vi "controlLaw_Integral_trackTraj.vi"(7 "ControlParams":T1={"umax"=3.0, "y_ref(k)"=0.0, "Ki"=0.0, "y(k) (from plant)"=0.0, "ND"=0, "NS"=0, "u_Kx_ref(k)"=0.0, "du_max"=3.0, "NS_obs"=0, "NS_control"=0} {"du_max" format="%#_13g"; "u_Kx_ref(k)" format="%#_13g"; "Ki" format="%#_13g"; "y_ref(k)" format="%#_13g"; "umax" format="%#_13g"}, 8 "x^(k)":sgl[](array[numeric])=[0.0, 0.0, 0.0, 0.0, 0.0, 0.0, 0.0, 0.0, 0.0, 0.0, 0.0, 0.0, 0.0, 0.0, 0.0, 0.0, 0.0, 0.0, 0.0, 0.0, 0.0, 0.0, 0.0, 0.0, 0.0]) -> (0 "x^(k+1) = Ax + Bu + Lye":sgl[](array[numeric]), 3 "u(k) (saturated)":sgl)   [LabVIEW 2017]
uses:
  controls/controlParams_tracktraj.ctl
  <vilib>/Platform/TimedLoop/XDataNode/timing_clust.ctl
  <vilib>/Platform/TimedLoop/XDataNode/nitl_modes.ctl
  <vilib>/Platform/TimedLoop/XDataNode/wakeup.ctl
  <vilib>/rvi/DataTransferAndStorage/Container/Common/niFpgaContainerExecOnDevCompGetState.vi
  <vilib>/rvi/Emulation/niFpgaEmulationIsFPGAContextNoSignature.vi
  <vilib>/rvi/DataTransferAndStorage/Container/Common/niFpgaContainerGetUniqueNameForEmu.vi
  <vilib>/rvi/Memory/Memory_Emulation/niFpgaMemoryEmulationCacheClearOnFirstRun.vi
  <vilib>/rvi/Memory/Memory_Emulation/nirvimemoryEmulationManagerCache_MakeExclusive.vi
  <vilib>/rvi/Memory/Memory_Emulation/niFpgaMemoryEmulationValidateCache.vi
  <vilib>/rvi/Memory/Memory_Emulation/nirvimemoryEmulationManagerCache_InsertValue.vi
  <vilib>/Utility/error.llb/Clear Errors.vi
  <vilib>/rvi/Memory/Memory_Emulation/nirvimemoryEmulationManagerCache_ReleaseExclusive.vi
  <vilib>/rvi/Memory/Memory_Emulation/nirvimemoryEmulationManagerCache_GetValue.vi
  <vilib>/rvi/Memory/Memory_Emulation/nirvimemoryEmulationManagerCache_SetValue.vi
  <vilib>/rvi/Emulation/niFpgaProcessEmulError.vi
  <vilib>/rvi/Emulation/niFpgaSctlEmulationGetInTimedLoop.vi
  <vilib>/rvi/Emulation/niFpgaEmulationReportErrorSimple.vi
  <vilib>/rvi/Emulation/niFpgaGetClockAttributes.vi
  <vilib>/rvi/Emulation/niFpgaCriticalErrorInLSC.vi
  <vilib>/Platform/TimedLoop/XDataNode/XDataNode.xnode
  <vilib>/rvi/DataTransferAndStorage/Container/XNode/niFpgaContainer.xnode
  <vilib>/rvi/DataTransferAndStorage/Register/Emulation/niFpgaRegisterEmulationRefIn.vi
  <vilib>/Platform/TimedLoop/XDataNode/XDNodeRunTimeDep.lvlib
panel:
  out "u = -Kx + Nbar*r":sgl format="%#_13g"
  out "-K*x(k)":sgl format="%#_13g"
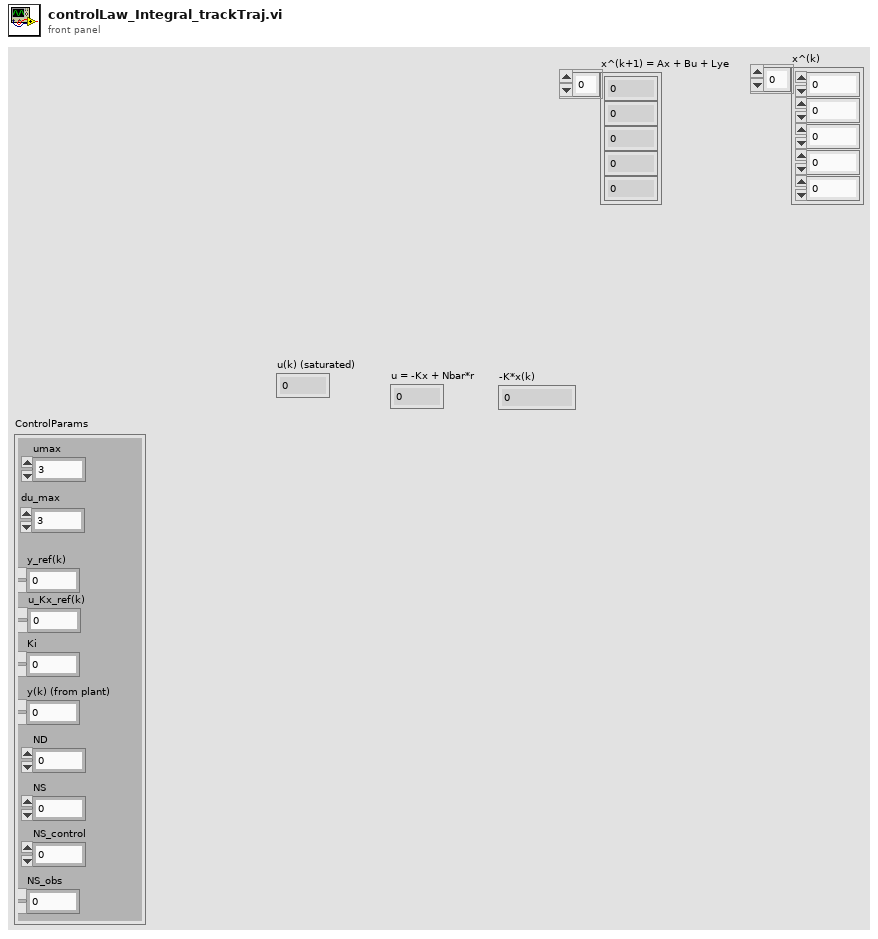
[diagram p1: front panel]
types:
  T1 = typedef "controlParams_tracktraj.ctl" = cluster{"umax":sgl, "y_ref(k)":sgl, "Ki":sgl, "y(k) (from plant)":sgl, "ND":i16, "NS":i16, "u_Kx_ref(k)":sgl, "du_max":sgl, "NS_obs":i16, "NS_control":i16}
  T2 = typedef "XDNodeRunTimeDep.lvlib/timing_clust.ctl" = cluster{"Expected End [f-1]":u64, "Actual End [f-1]":u64, "Finished Late? [f-1]":bool, "Expected End [i-1]":u64, "Actual End [i-1]":u64, "Finished Late? [i-1]":bool, "Expected Start [i]":u64, "Actual Start [i]":u64, "Expected Start [f]":u64, "Actual Start [f]":u64, "Source Name":string, "Structure Name":string, "Period":i64, "Deadline":i64, "Offset":i64, "Start":i64, "Priority":i32, "Timeout":i32, "Mode":T3, "Wakeup Reason":T4, "Error":errorcluster, "Source Type":string, "Secondary Source Type":string, "Global End Time":u64, "Global Start Time":u64, "Frame Duration":u64, "Iteration Duration":u64, "Assigned CPU":i32, "I/O Scan Engine Mode":u32}
  T3 = typedef "XDNodeRunTimeDep.lvlib/nitl_modes.ctl" = enum32{"No Change", "Process missed periods, maintain original phase", "Discard missed periods, maintain original phase", "Process missed periods, ignore original phase", "Discard missed periods, ignore original phase"}
  T4 = typedef "XDNodeRunTimeDep.lvlib/wakeup.ctl" = enum32{"Normal", "Aborted", "Asynchronous wakeup", "Timing source error", "Timed loop error", "Timeout"}
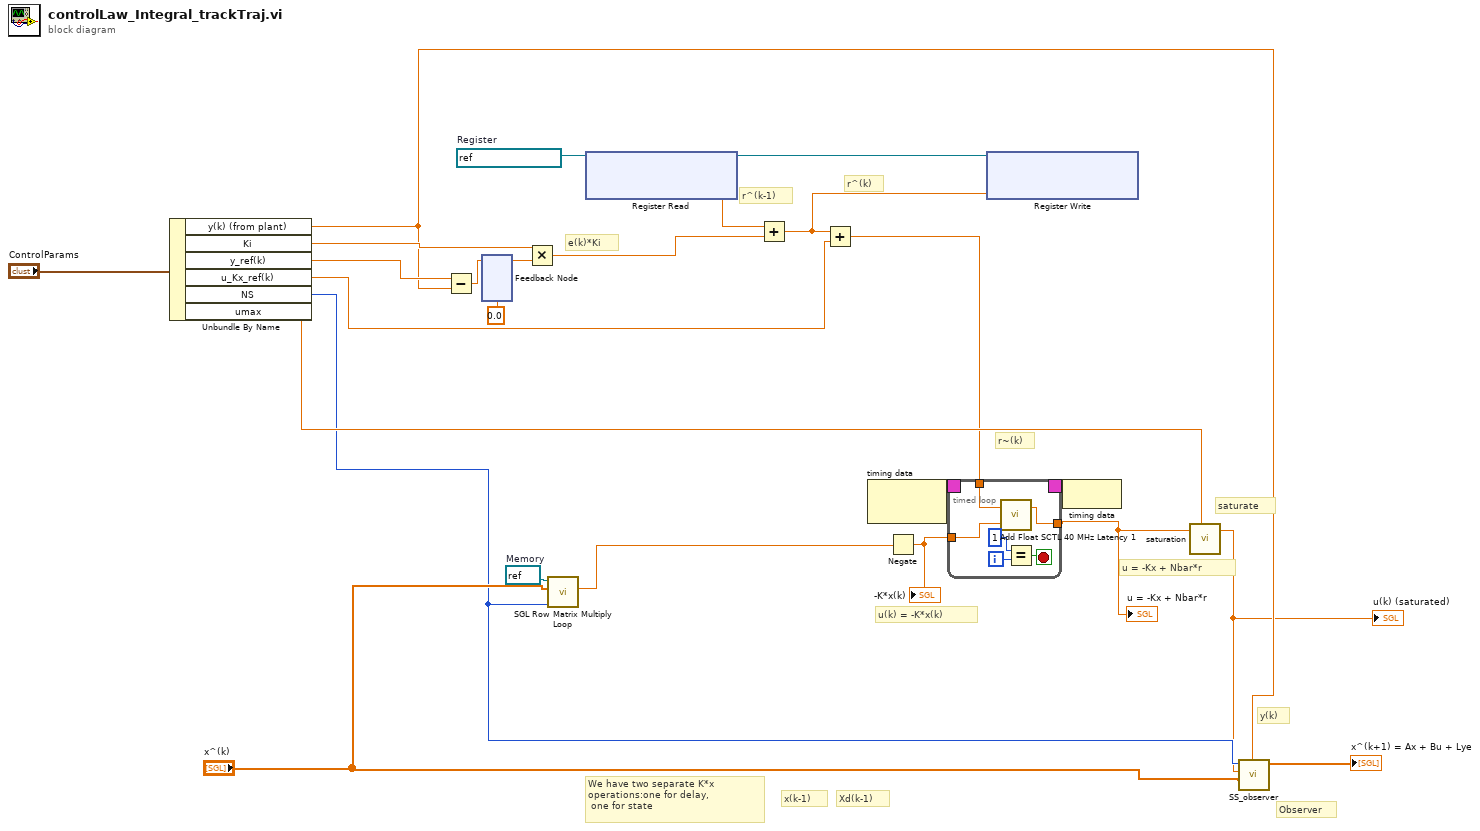
[diagram p0: block diagram]
diagram:
  w16 = refnum<k21> "accumulator"  # Register
  w21 = refnum<k21> "K"  # Memory
  # "y(k)"
  # "Xd(k-1)"
  # "x(k-1)"
  # "r^(k)"
  # "r^(k-1)"
  # "e(k)*Ki"
  # "r~(k)"
  # "We have two separate K*x\noperations:one for delay,\n one for state"
  # "saturate"
  # "u = -Kx + Nbar*r"
  # "u(k) = -K*x(k)"
  # "Observer"
  n1 = Unbundle By Name("ControlParams") -> ("y(k) (from plant)"=w7:sgl, "Ki"=w15:sgl, "y_ref(k)"=w14:sgl, "u_Kx_ref(k)"=w9:sgl, "NS"=w4:i16, "umax"=w13:sgl)
  n2 = Subtract(x=w14, y=w7) -> (x-y=w11:sgl)
  n3 = feedback #1(sgl 0.0) -> (w12:sgl)
  n4 = feedback-in #1(w11) -> ()
  n5 = Multiply(x=w15, y=w12) -> (x*y=w18:sgl)
  n6 = call "SGL Row Matrix Multiply Loop.vi"("NS"=w4, "X"="x^(k)", "Refnum in"=w21) -> ("Numeric"=w2:sgl)  [unwired: 8 in]
  n7 = xnode ("Register Read")("Register In"=w16) -> ("Data"=w19:sgl, "Register Out"=w20:refnum<k21>)
  n8 = Add(x=w19, y=w18) -> (x+y=w17:sgl)
  n9 = Add(x=w17, y=w9) -> (x+y=w8:sgl)
  n10 = node-c288() -> (w25:T2)  [unwired: 1 in]
  n11 = Negate(x=w2) -> (-x=w22:sgl)
  "-K*x(k)" <- w22
  n12 = timed-loop {
    timing: w25 -> [_]
    timing-out: [_] -> w24
    tunnel: w8 -> [w31]
    tunnel: w22 -> [w30]
    tunnel: [w26] -> w23
    i -> [w27]
    stop <- w29 stop-if-true
    n13 = call "Add Float SCTL 40 MHz Latency 1.vi"("y"=w30, "x"=w31) -> ("x[k-1]+y[k-1]"=w26:sgl)  [unwired: 1 out]
    n14 = Equal?(x=i16 1, y=w27) -> (x = y?=w29:bool)
  }
  "u = -Kx + Nbar*r" <- w23
  n15 = xnode ("Register Write")("Data"=w17, "Register In"=w20) -> ()  [unwired: 1 out]
  n16 = node-c288(w24) -> ()
  n17 = call "saturation.vi"("uMax"=w13, "signal in"=w23) -> ("signal out"=w3:sgl)  [unwired: 9 in]
  "u(k) (saturated)" <- w3
  n18 = call "SS_observer.vi"("y(k)"=w7, "X"="x^(k)", "u(k)"=w3, "NS"=w4) -> ("Ax + Bu + Lye"=→"x^(k+1) = Ax + Bu + Lye":sgl[])  [unwired: 7 in]
